vi "SetObservers.vi"(8 "error in (no error)":errorcluster, 10 "Observers":refnum<class "Observer.lvclass">[](array[class]), 11 "Observable in":refnum<class "Observable.lvclass">) -> (0 "error out":errorcluster, 3 "Observable out":refnum<class "Observable.lvclass">)   [LabVIEW 2020, in "Observable.lvclass"]
uses:
  Observable.lvclass
  Observer/Observer.lvclass
  Observable.lvclass/Observable.ctl
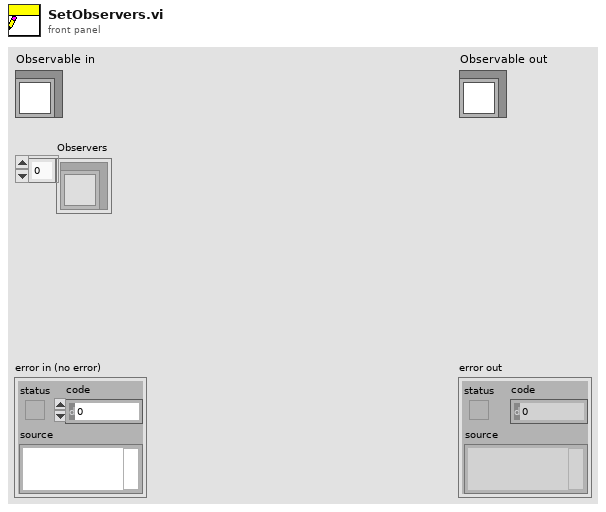
[diagram p1: front panel]
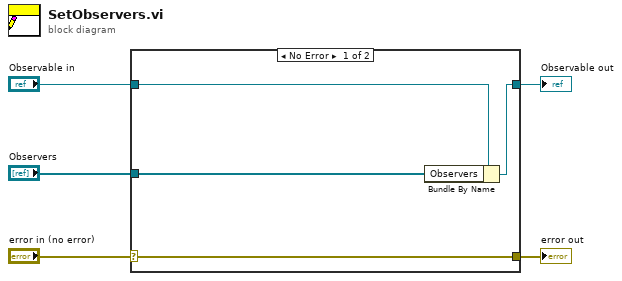
[diagram p0: block diagram]
diagram:
  n1 = case shown="No Error" "error in (no error)" {
    selector: "error in (no error)" -> [w9 w10]
    tunnel: [w9 w10] -> w4
    tunnel: [w7 w11] -> w2
    tunnel: "Observable in" -> [w8 w11]
    tunnel: "Observers" -> [w6 _]
    frame No Error {
      n2 = Bundle By Name(cluster=w8, "Observers"=w6) -> (w7:refnum<class "Observable.lvclass">)
    }
    frame Error {
    }
  }
  "error out" <- w4
  "Observable out" <- w2
